vi "PCE-Archive.vi"(7 "Nouvelle Commande":T2, 8 "MaxLength":i32, 11 "CmdDone IN":T1(array[cluster]) caption="Commandes Effectués") -> (3 "CmdDone OUT":T1(array[cluster]) caption="Commandes Sortantes")   [LabVIEW 2011]
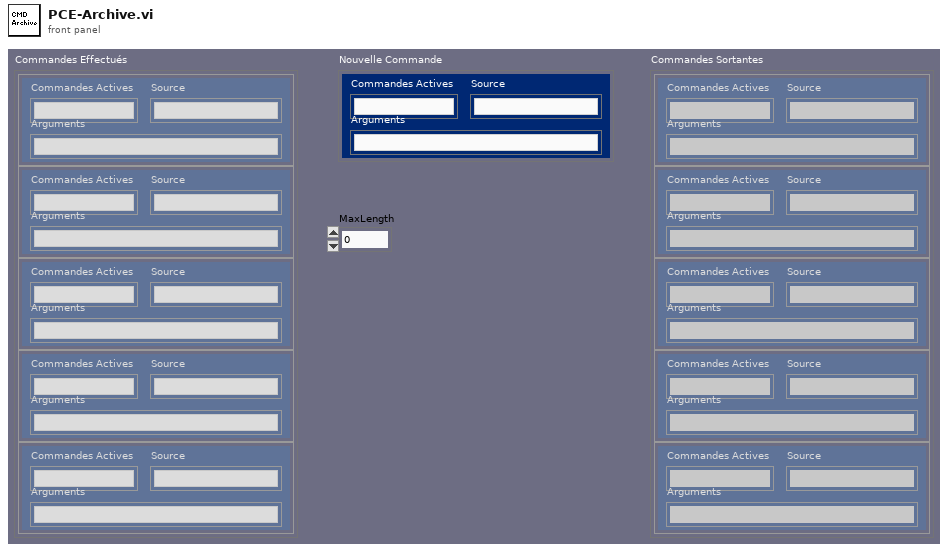
[diagram p1: front panel]
types:
  T1 = cluster{"CmdAct":string, "CmdArgs":string, "Source":string}[]
  T2 = cluster{"CmdAct":string, "CmdArgs":string, "Source":string}
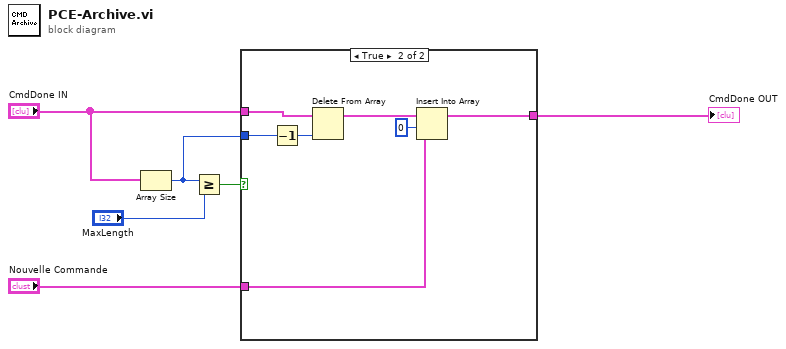
[diagram p0: block diagram]
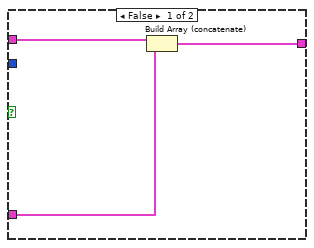
[diagram p2: hidden frame]
diagram:
  n1 = Array Size(array="CmdDone IN") -> (size(s)=w1:i32)
  n2 = Greater Or Equal?(x=w1, y="MaxLength") -> (x >= y?=w4:bool)
  n3 = case shown="True" w4 {
    tunnel: "CmdDone IN" -> [w9 w16]
    tunnel: "Nouvelle Commande" -> [w8 w11]
    tunnel: [w7 w14] -> w2
    tunnel: w1 -> [_ w13]
    frame False {
      n4 = Build Array (concatenate)(w9, w8) -> (w7:T1)
    }
    frame True {
      n5 = Decrement(x=w13) -> (x-1=w12:i32)
      n6 = Delete From Array(array=w16, index=w12) -> (array with subset deleted=w15:T1)  [unwired: 1 in, 1 out]
      n7 = Insert Into Array(array=w15, index=0, new element=w11) -> (w14:T1)
    }
  }
  "CmdDone OUT" <- w2
